vi "PBcard_load.vi"(0 "PulseBlaster\nVLIW Array":T1(array[cluster])=[{"Output Bits"=4739583, "Data Field"=0, "OP Code"=1, "Delay Count"=99999999997}] {"OP Code" format="%.0x"; "Output Bits" format="%x"}, 1 "Bytes/Word":u8=10, 2 "Memory":bool, 3 "error in":errorcluster, 4 "Select Board Indicator":i32) -> (7 "error out":errorcluster)   [LabVIEW 2013, in "PulseBlaster.lvlib"]
doc: "PBcard_load: \nThis vi \n1) resets the PB, (consists of 4 steps)\n2) writes an array of VLIW's (very long instruction word) to the PB memory\n3) sends \"program finished\".\nAfter completion, a \"start\" command to the PB will make it run the programmed sequence. \n\nThe VLIW is implemented as a cluster of four integers (24bit, 20bit, 4bit, 32bit).\n\nNOTE: NO ERROR CHECKING IS PERFORMED. Error checking is supposedly taken care of before the VLIW array image is made, for example by Add_VLIW, which writes a PulseBlaster command to an array in memory. An"
uses:
  PulseBlaster.lvlib
panel:
  # "External"
  # "Internal"
  # "(24 bits)"
  # "(20 bits)"
  # "(4 bits)"
  # "(32 bits)"
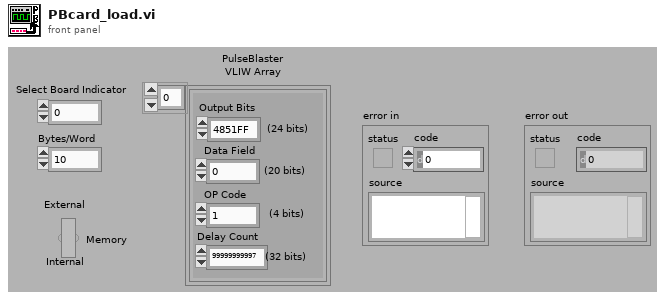
[diagram p1: front panel]
types:
  T1 = cluster{"Output Bits":u32, "Data Field":u32, "OP Code":u8, "Delay Count":u64}[]
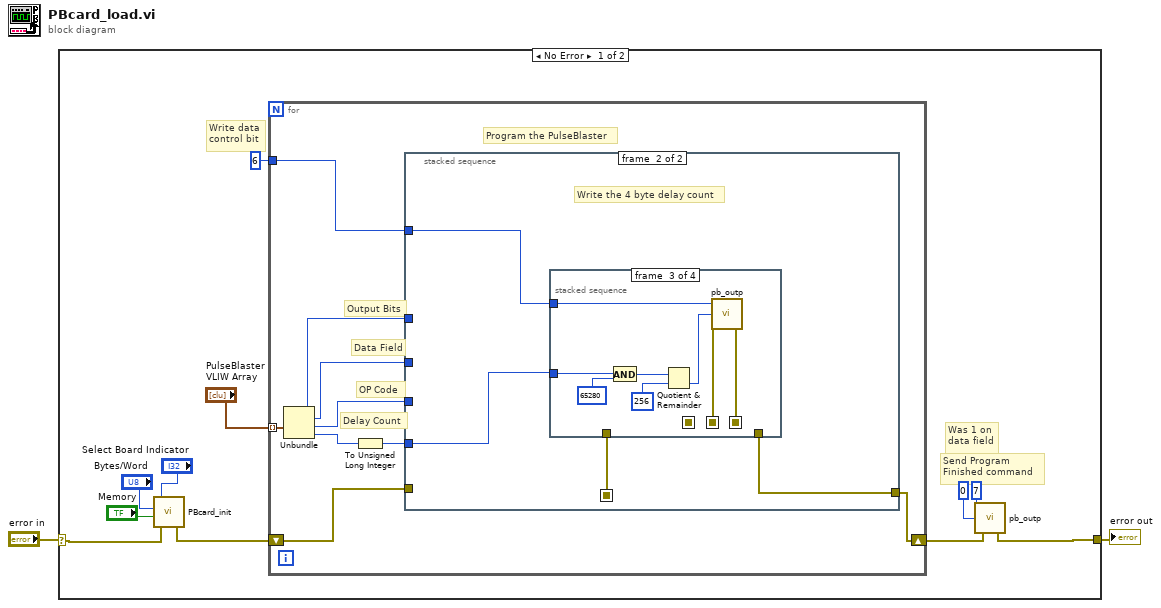
[diagram p0: block diagram]
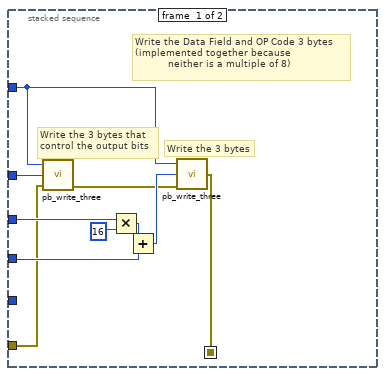
[diagram p2: hidden frame]
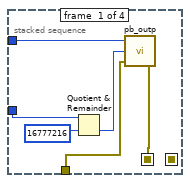
[diagram p3: hidden frame]
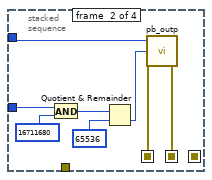
[diagram p4: hidden frame]
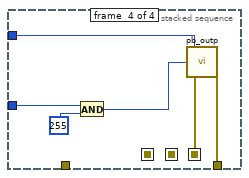
[diagram p5: hidden frame]
diagram:
  n1 = case shown="No Error" "error in" {
    selector: "error in" -> [w13 w65]
    tunnel: [w10 w65] -> w1
    frame No Error {
      # "Was 1 on\ndata field"
      # "Send Program\nFinished command"
      # "Write data\ncontrol bit"
      n2 = call "PBcard_init.vi"("error in (no error)"=w13, "Memory"="Memory", "Bytes/Word"="Bytes/Word", "Select Board\nIndicator"="Select Board Indicator") -> ("error out"=w12:errorcluster)
      n3 = for {
        tunnel: u8 6 -> [w22]
        tunnel: "PulseBlaster\nVLIW Array" -> [w17] mode=indexing
        shift-right: [w15] -> w11
        shift-left: w12 -> [w16]
        # "Program the PulseBlaster"
        # "Delay Count"
        # "OP Code"
        # "Data Field"
        # "Output Bits"
        n4 = Unbundle(w17) -> ("Output Bits"=w21:u32, "Data Field"=w20:u32, "OP Code"=w19:u8, "Delay Count"=w18:u64)
        n5 = To Unsigned Long Integer(number=w18) -> (unsigned 32bit integer=w14:u32)
        n6 = stacked-sequence {
          seq-local: [w23 _] -> [_ w34]
          tunnel: w21 -> [w26 _]
          tunnel: w20 -> [w32 _]
          tunnel: w19 -> [w30 _]
          tunnel: w22 -> [w27 w35]
          tunnel: w14 -> [_ w36]
          tunnel: w16 -> [w25 _]
          tunnel: [_ w33] -> w15
          frame #0 {
            # "Write the 3 bytes that \ncontrol the output bits"
            # "Write the 3 bytes"
            # "Write the Data Field and OP Code 3 bytes\n(implemented together because \n           neither is a multiple of 8)"
            n7 = call "pb_write_three.vi"("error in (no error)"=w25, "8-bit data"=w26, "8-bit address offset"=w27) -> ("error out"=w24:errorcluster)
            n8 = Multiply(x=w32, y=u32 16) -> (x*y=w29:u32)
            n9 = Add(x=w29, y=w30) -> (x+y=w28:u32)
            n10 = call "pb_write_three.vi"("error in (no error)"=w24, "8-bit data"=w28, "8-bit address offset"=w27) -> ("error out"=w23:errorcluster)
          }
          frame #1 {
            # "Write the 4 byte delay count"
            n11 = stacked-sequence {
              seq-local: [w37 _ _ _] -> [_ w44 _ _]
              seq-local: [_ w43 _ _] -> [_ _ w52 _]
              seq-local: [_ _ w51 _] -> [_ _ _ w60]
              tunnel: w36 -> [w41 w47 w55 w63]
              tunnel: w35 -> [w40 w46 w54 w62]
              tunnel: w34 -> [w38 _ _ _]
              tunnel: [_ _ _ w59] -> w33
              frame #0 {
                n12 = Quotient & Remainder(x=w41, y=u32 16777216) -> (floor(x/y)=w39:u32)  [unwired: 1 out]
                n13 = call "pb_outp.vi"("error in (no error)"=w38, "8-bit data"=w39, "8-bit address offset"=w40) -> ("error out"=w37:errorcluster)
              }
              frame #1 {
                n14 = And(x=w47, y=u32 16711680) -> (x .and. y?=w48:u32)
                n15 = Quotient & Remainder(x=w48, y=u32 65536) -> (floor(x/y)=w45:u32)  [unwired: 1 out]
                n16 = call "pb_outp.vi"("error in (no error)"=w44, "8-bit data"=w45, "8-bit address offset"=w46) -> ("error out"=w43:errorcluster)
              }
              frame #2 {
                n17 = And(x=w55, y=u32 65280) -> (x .and. y?=w56:u32)
                n18 = Quotient & Remainder(x=w56, y=u32 256) -> (floor(x/y)=w53:u32)  [unwired: 1 out]
                n19 = call "pb_outp.vi"("error in (no error)"=w52, "8-bit data"=w53, "8-bit address offset"=w54) -> ("error out"=w51:errorcluster)
              }
              frame #3 {
                n20 = And(x=w63, y=u32 255) -> (x .and. y?=w61:u32)
                n21 = call "pb_outp.vi"("error in (no error)"=w60, "8-bit data"=w61, "8-bit address offset"=w62) -> ("error out"=w59:errorcluster)
              }
            }
          }
        }
      }
      n22 = call "pb_outp.vi"("error in (no error)"=w11, "8-bit data"=u8 0, "8-bit address offset"=u8 7) -> ("error out"=w10:errorcluster)
    }
    frame Error {
    }
  }
  "error out" <- w1
